vi "DG535.set outputs.vi"(0 "i ref in":refnum<vi>, 1 "output":i32(ring) items=["T0", "A", "B", "AB", "C", "D", "CD"], 2 "mode":i32(ring) items=["TTL", "NIM", "ECL", "VAR"], 3 "amplitude":i32=1 min=-3 max=4, 4 "offset":i32 min=-3 max=4, 5 "error in (no error)":errorcluster, 6 "set":bool, 7 "inversion":bool, 9 "load":bool) -> (14 "i ref out":refnum<vi>, 19 "error out":errorcluster)   [LabVIEW 2014, in "DG535.lvlib"]
doc: "This vi can be used to setup the outputs signal parameters. Select a channel to set with the \"output\" control, define all its parameters then press the \"Set\" control to send the data to the device."
uses:
  DG535.lvlib
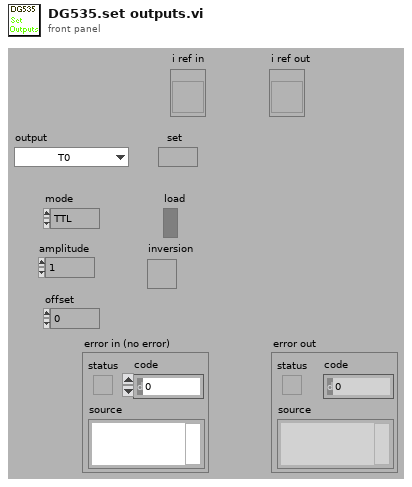
[diagram p1: front panel]
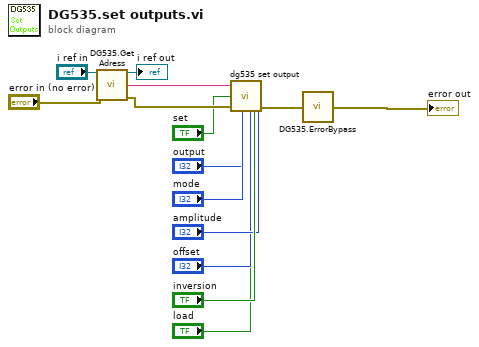
[diagram p0: block diagram]
diagram:
  n1 = call "DG535.Get Adress.vi"("i ref in"="i ref in", "error in (no error)"="error in (no error)") -> ("i ref out"=→"i ref out":refnum<vi>, "address"=w10:string, "error out"=w11:errorcluster)  [unwired: 10 in, 1 out]
  n2 = call "dg535 set output.vi"("GPIB address"=w10, "output"="output", "set"="set", "error in"=w11, "mode"="mode", "offset"="offset", "amplitude"="amplitude", "inversion"="inversion", "load"="load") -> ("error out"=w9:errorcluster)
  n3 = call "DG535.ErrorBypass.vi"("error in (no error)"=w9) -> ("error out"=→"error out":errorcluster)  [unwired: 14 in]
